vi "Configure MCCW Power and Phase.vi"(8 "error in (no error)":errorcluster, 9 "Phase":dbl[](array[numeric]), 10 "Power":dbl[](array[numeric]), 11 "VSG-SMBV in":refnum<class "VSG-SMBV.lvclass">) -> (0 "error out":errorcluster, 3 "VSG-SMBV out":refnum<class "VSG-SMBV.lvclass">)   [LabVIEW 2020, in "VSG-SMBV.lvclass"]
doc: "Configures the relative power level and phase for each carrier"
uses:
  VSG-SMBV.lvclass
  C:/Sandbox/RF Bench/Source Code/WiSpry Test Framework/Instruments/Instrument.lvclass
  Instrument.lvclass/Instrument.ctl
  Instrument.lvclass
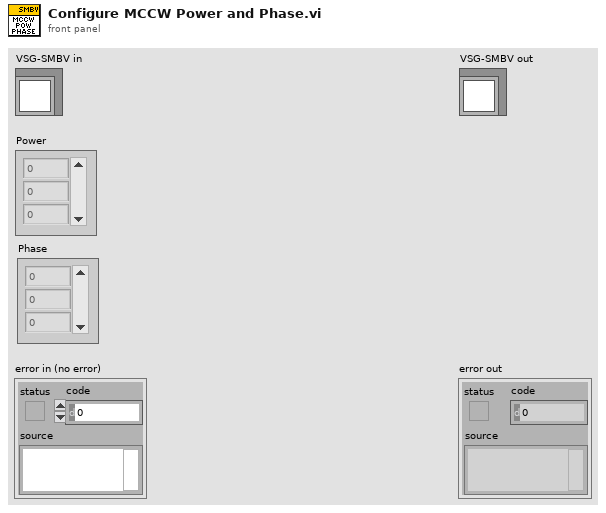
[diagram p1: front panel]
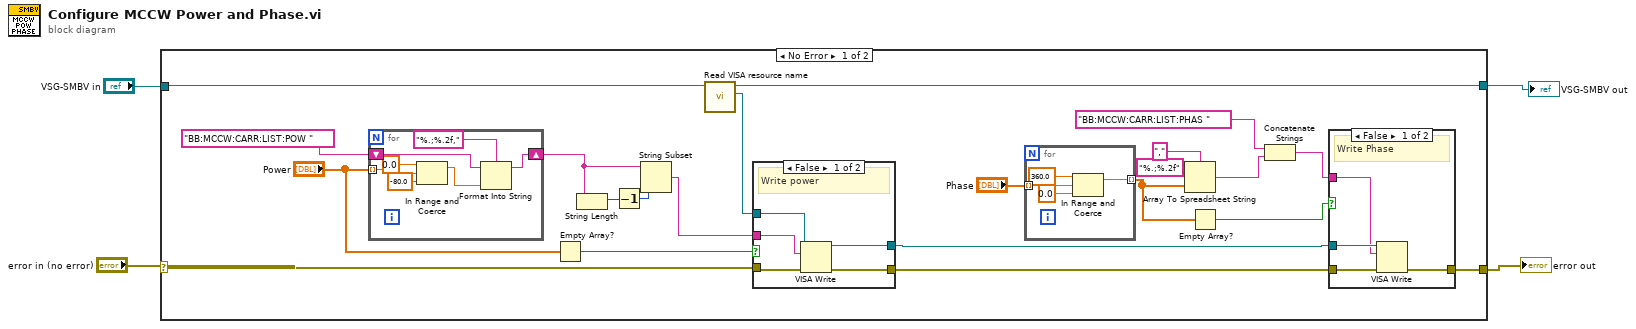
[diagram p0: block diagram]
diagram:
  n1 = case shown="No Error" "error in (no error)" {
    selector: "error in (no error)" -> [w18 w50]
    tunnel: "VSG-SMBV in" -> [w26 w51]
    tunnel: [w25 w51] -> w2
    tunnel: [w8 w50] -> w1
    frame No Error {
      n2 = for {
        tunnel: "Power" -> [w46] mode=indexing
        shift-right: [w47] -> w22
        shift-left: "BB:MCCW:CARR:LIST:POW " ("string") -> [w49]
        n3 = In Range and Coerce(upper limit=0.0, x=w46, lower limit=-80.0) -> (coerced(x)=w45:dbl)  [unwired: 1 out]
        n4 = Format Into String(format string="%.;%.2f,", initial string=w49, w45) -> (resulting string=w47:string)  [unwired: 1 in, 1 out]
      }
      n5 = Empty Array?(array="Power") -> (empty?=w19:bool)
      n6 = String Length(string=w22) -> (length=w23:i32)
      n7 = Decrement(x=w23) -> (x-1=w21:i32)
      n8 = String Subset(string=w22, length (rest)=w21) -> (substring=w16:string)  [unwired: 1 in]
      n9 = call "Read VISA resource name.vi"("Instrument in"=w26) -> ("VISA resource name"=w17:refnum<visa-resource-name>, "Instrument out"=w25:refnum<class "VSG-SMBV.lvclass">)  [unwired: 9 in]
      n10 = case shown="False" w19 {
        tunnel: w18 -> [w40 w41]
        tunnel: w17 -> [w38 w42]
        tunnel: w16 -> [w39 _]
        tunnel: [w37 w42] -> w10
        tunnel: [w36 w41] -> w9
        frame False {
          # "Write power"
          n11 = VISA Write(VISA resource name=w38, write buffer=w39, error in (no error)=w40) -> (VISA resource name out=w37:refnum<visa-resource-name>, error out=w36:errorcluster)  [unwired: 1 out]
        }
        frame True {
        }
      }
      n12 = for {
        tunnel: "Phase" -> [w35] mode=indexing
        tunnel: [w32] -> w12 mode=indexing
        n13 = In Range and Coerce(upper limit=360.0, x=w35, lower limit=0.0) -> (coerced(x)=w32:dbl)  [unwired: 1 out]
      }
      n14 = Array To Spreadsheet String(delimiter (Tab)=",", array=w12, 3:"%.;%.2f" ("format string")) -> (spreadsheet string=w6:string)
      n15 = Empty Array?(array=w12) -> (empty?=w11:bool)
      n16 = Concatenate Strings("BB:MCCW:CARR:LIST:PHAS ", w6) -> (w5:string)
      n17 = case shown="False" w11 {
        tunnel: w10 -> [w30 _]
        tunnel: w5 -> [w29 _]
        tunnel: w9 -> [w28 w31]
        tunnel: [w27 w31] -> w8
        frame False {
          # "Write Phase"
          n18 = VISA Write(VISA resource name=w30, write buffer=w29, error in (no error)=w28) -> (error out=w27:errorcluster)  [unwired: 2 out]
        }
        frame True {
        }
      }
    }
    frame Error {
    }
  }
  "error out" <- w1
  "VSG-SMBV out" <- w2
